vi "Read Name.vi"(11 "Person In":refnum<class "Person.lvclass">) -> (2 "Name":string, 3 "Person Out":refnum<class "Person.lvclass">)   [LabVIEW 2018, in "Person.lvclass"]
uses:
  Person.lvclass
  Person.lvclass/Person.ctl
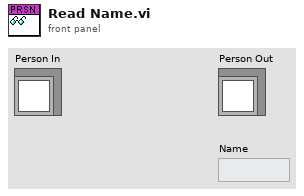
[diagram p1: front panel]
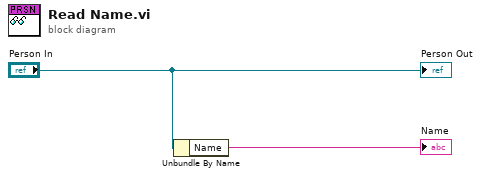
[diagram p0: block diagram]
diagram:
  n1 = Unbundle By Name("Person In") -> ("Name"=→"Name":string)
  "Person Out" <- "Person In"
